vi "datalogging_sub.vi"(7 "Filename":string="RedData.dat", 10 "Encoder Vals":i32[](array[numeric]), 11 "NXT/EV3 In":T1) -> (3 "NXT/EV3 Out":T1)   [LabVIEW 2012, in "Mecanum Drive.lvrbt"]
uses:
  Mecanum Drive.lvrbt
  <vilib>/NXT/Subs/LVHSConnector.ctl
  <vilib>/NXT/LegoClasses/BrickReference/BrickReference.lvclass
  <vilib>/NXT/NXTIO Xnodes/NXTIONodeSubVIs/LEGOStopAllMotors.vi
  <vilib>/NXT/NXTIO Xnodes/NXTIONodeSubVIs/LEGOMoveAllMotors.vi
  <vilib>/NXT/NXTIO Xnodes/NXTIOXNode/NXTIO.xnode
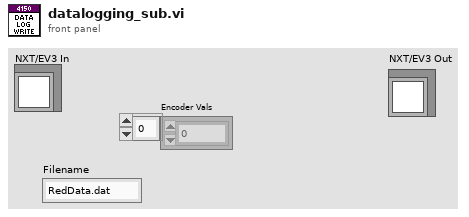
[diagram p1: front panel]
types:
  T1 = typedef "LVHSConnector.ctl" = refnum<class "BrickReference.lvclass">
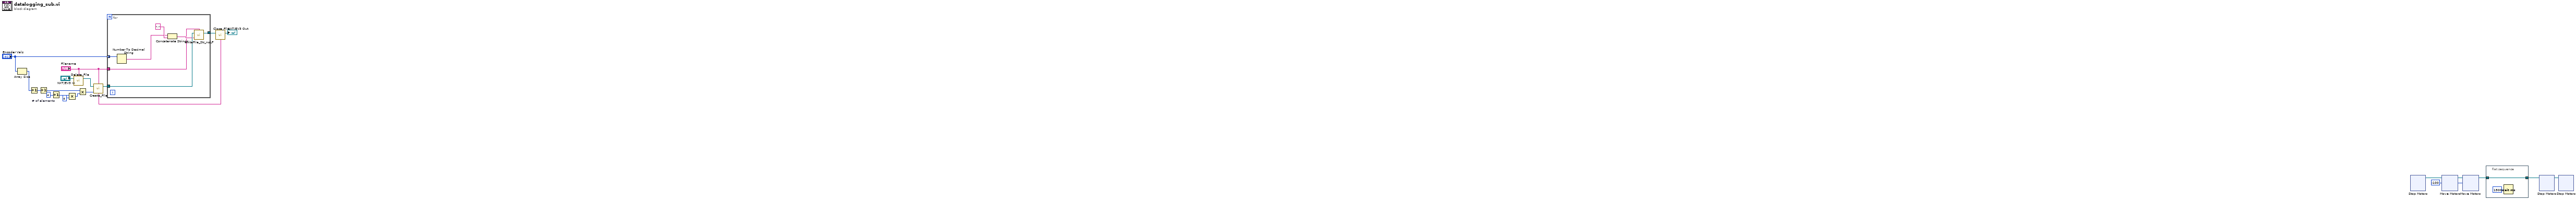
[diagram p0: block diagram]
diagram:
  w13 = 4  # # of elements
  w21 = i8 -100 ("Power/Speed 1")
  n1 = Array Size(array="Encoder Vals") -> (size(s)=w6:i32)
  n2 = Increment(x=w6) -> (x+1=w14:i32)
  n3 = Increment(x=w14) -> (x+1=w9:i32)
  n4 = Increment(x=w13) -> (x+1=w12:i32)
  n5 = Multiply(x=w12, y=u32 4) -> (x*y=w11:u32)
  n6 = call <vilib>:"Delete_File.vi"("NXT/EV3"="NXT/EV3 In", "Filename"="Filename") -> ("NXT/EV3"=w8:T1)  [unwired: 2 in]
  n7 = Multiply(x=w9, y=w11) -> (x*y=w15:u32)
  n8 = call <vilib>:"Create_File.vi"("File Size (256)"=w15, "NXT/EV3"=w8, "Filename"="Filename") -> ("NXT/EV3"=w5:T1)  [unwired: 1 out]
  n9 = for {
    tunnel: "Encoder Vals" -> [w24] mode=indexing
    tunnel: w5 -> [w28]
    tunnel: "Filename" -> [w23]
    tunnel: [w27] -> w4
    n10 = Number To Decimal String(number=w24) -> (decimal integer string=w22:string)  [unwired: 1 in]
    n11 = Concatenate Strings(w22, "," ("string")) -> (w26:string)
    n12 = call <vilib>:"WriteFile_Str_noLF.vi"("String"=w26, "NXT/EV3"=w28, "Filename"=w23) -> ("NXT/EV3"=w27:T1)  [unwired: 1 in]
  }
  n13 = call <vilib>:"Close_File.vi"("NXT/EV3"=w4, "Filename"="Filename") -> ("NXT/EV3"=→"NXT/EV3 Out":T1)  [unwired: 2 in]
  n14 = xnode "Stop Motors"() -> ("NXT/EV3"=w16:T1)  [unwired: 2 in]
  n15 = xnode "Move Motors"("Power/Speed 1"=w21, "NXT/EV3"=w16) -> ("NXT/EV3"=w20:T1)  [unwired: 1 in]
  n16 = xnode "Move Motors"("Power/Speed 1"=w21, "NXT/EV3"=w20) -> ("NXT/EV3"=w17:T1)  [unwired: 1 in]
  n17 = flat-sequence {
    tunnel: [w29] -> w19
    tunnel: w17 -> [w29]
    frame #0 {
      n18 = Wait (ms)(milliseconds to wait=u32 1500) -> ()  [unwired: 1 out]
    }
  }
  n19 = xnode "Stop Motors"("NXT/EV3"=w19) -> ("NXT/EV3"=w18:T1)  [unwired: 1 in]
  n20 = xnode "Stop Motors"("NXT/EV3"=w18) -> ()  [unwired: 1 in, 1 out]
